vi "Get Uncovered Diagrams.vi"(8 "error in (no error)":errorcluster, 10 "VI Path":path, 11 "CodeCoverage in":refnum<class "Code Coverage.lvclass">) -> (0 "error out":errorcluster, 2 "Uncovered Diagrams":refnum<vi>[](array[refnum]), 3 "CodeCoverage out":refnum<class "Code Coverage.lvclass">)   [LabVIEW 2017, in "Code Coverage.lvclass"]
doc: "Returns the code coverage percentage for a given VI."
uses:
  Code Coverage.lvclass
  Code Coverage.lvclass/Code Coverage.ctl
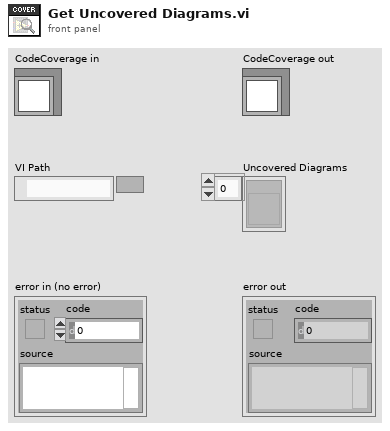
[diagram p1: front panel]
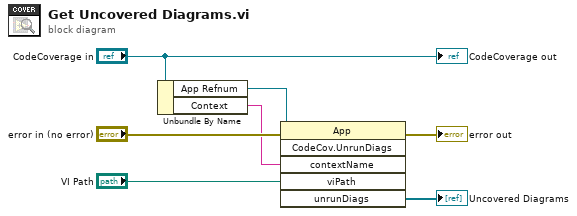
[diagram p0: block diagram]
diagram:
  n1 = Unbundle By Name("CodeCoverage in") -> ("App Refnum"=w3:refnum<vi>, "Context"=w1:string)
  n2 = invoke class="App" method="CodeCov.UnrunDiags"(reference=w3, error in="error in (no error)", "contextName"=w1, "viPath"="VI Path") -> (error out=→"error out":errorcluster, "unrunDiags"=→"Uncovered Diagrams":refnum<vi>[])  [unwired: 2 in, 4 out]
  "CodeCoverage out" <- "CodeCoverage in"
